vi "Dashboard Main for German stuff.vi"() -> ()   [LabVIEW 2013]
uses:
  <vilib>/Rock Robotics/WPI/DriverStation/WPI_DriverStationAllianceInfo.ctl
  <vilib>/Rock Robotics/WPI/Dashboard/WPI_DashboardLogging Global.vi
  <vilib>/Rock Robotics/WPI/Camera/WPI_CameraImageSize.ctl
  <vilib>/Rock Robotics/WPI/Camera/WPI_CameraSettings Read MJPG.ctl
panel:
  in  "Sudden Sound":bool
  in  "Oh Nein":bool
  out "Left Speed":dbl
  out "Right Speed":dbl
  in  "Precious":bool
  in  "Pokemon":bool
  in  "Yoda":bool
  in  "Alarm":bool
  in  "Scotty":bool
  in  "Hal":bool
  in  "Game over":bool
  in  "Gandalf":bool
  out "Teleop Time":dbl(slide) scale=0.0..150.0
  out "Right Power":dbl(slide) scale=-1.0..1.0
  out "Left Power":dbl(slide) scale=-1.0..1.0
  out "Shooter":u16(ring)
  out "Loader":u16(ring)
  out "Picture Information":u16(ring)
  in  "Camera view range":dbl=33.5 format="%#_13g"
  in  "Alliance 2":T1
  in  "Hot Side":dbl
  in  "Shooting Position Options":T2={TRUE, TRUE, TRUE, TRUE, TRUE, TRUE, TRUE, TRUE, TRUE, TRUE}
  out "Time Remaining":dbl(slide) scale=0.0..150.0
  in  "stop":bool
  out "Camera IP":string
  in  "DB Camera Config":bool
  out "Image Message":string="Timeout in Camera Communications"
  in  "Rec Mode":enum32{"Stop", "Record", "Playback"}(radio)
  out "Secondary Driver Camera":T3(plugin-control)
  out "Primary Driver Camera":T3(plugin-control)
  # "TeleOperated"
  # "Primary Driver Side"
  # "Secondary Driver Side"
  # "Autonomous"
  # "Checklist\n\n1: Is the robot plugged in?\n2: Is the robot turned on?\n3: Are the balls in the correct position?\n4: Set up Autonomous (shooting position options)"
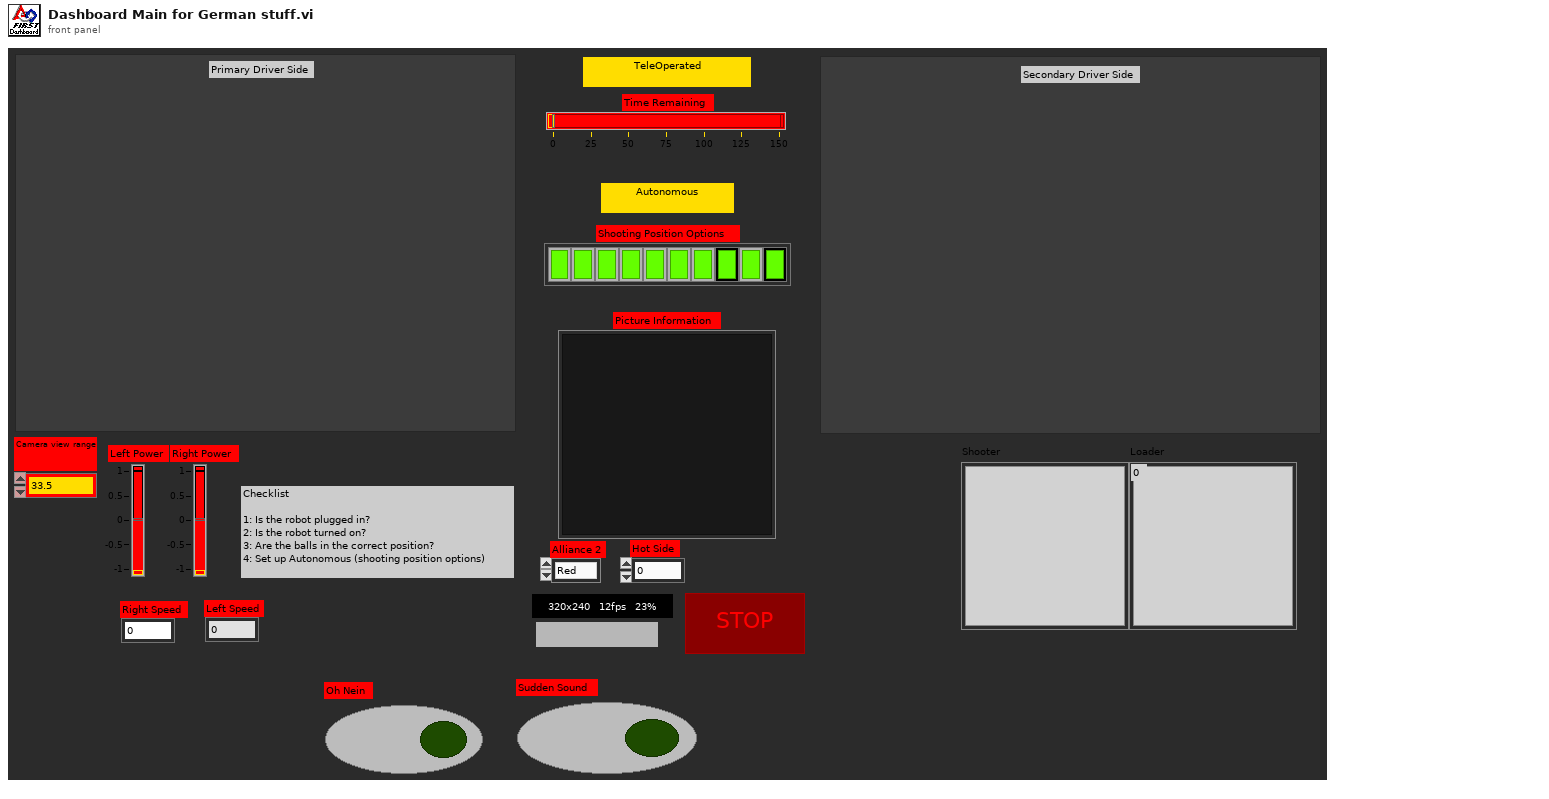
[diagram p1: front panel]
types:
  T1 = typedef "WPI_DriverStationAllianceInfo.ctl" = enum16{"Red", "Blue", "Invalid"}
  T2 = cluster{bool, bool, bool, bool, bool, bool, bool, bool, bool, bool}
  T3 = typedef "IMAQ Image.ctl" = refnum<image>
  T4 = cluster{"Left Power":dbl, "Right Power":dbl, "Shooter State":enum16{"Nothing", "Cocked", "Fire", "Load"}, "Loader State":enum16{"Loader Up", "Loader Down", "Ball In Possesion"}, "Auto Time":dbl, "Tele Time":dbl, "Driver":dbl, "Not Allowed":bool, "Right Speed":dbl, "Left Speed":dbl}
  T5 = enum16{"Loader Up", "Loader Down", "Ball In Possesion"}
  T6 = cluster{"Digital Inputs":bool[], "Digital Outputs":bool[]}
  T7 = cluster{"Competition mode":bool, "Robot Link":bool, "Autonomous":bool, "Enabled":bool, "E-Stop":bool, "Simulated":bool, "TestMode":bool, "Docked Window":bool}
  T8 = typedef "WPI_CameraSettings Read MJPG.ctl" = cluster{"fps":i32, "compression":i32, "Image Size":T9}
  T9 = typedef "WPI_CameraImageSize.ctl" = enum16{"640x480", "320x240", "160x120"}
  T10 = cluster{"Hue":dbl, "Saturation":dbl, "Luminance":dbl, "Hue Margin":dbl}
  T11 = typedef "Image Type" = u32
  T12 = cluster{"Left":i32, "Top":i32, "Right":i32, "Bottom":i32}
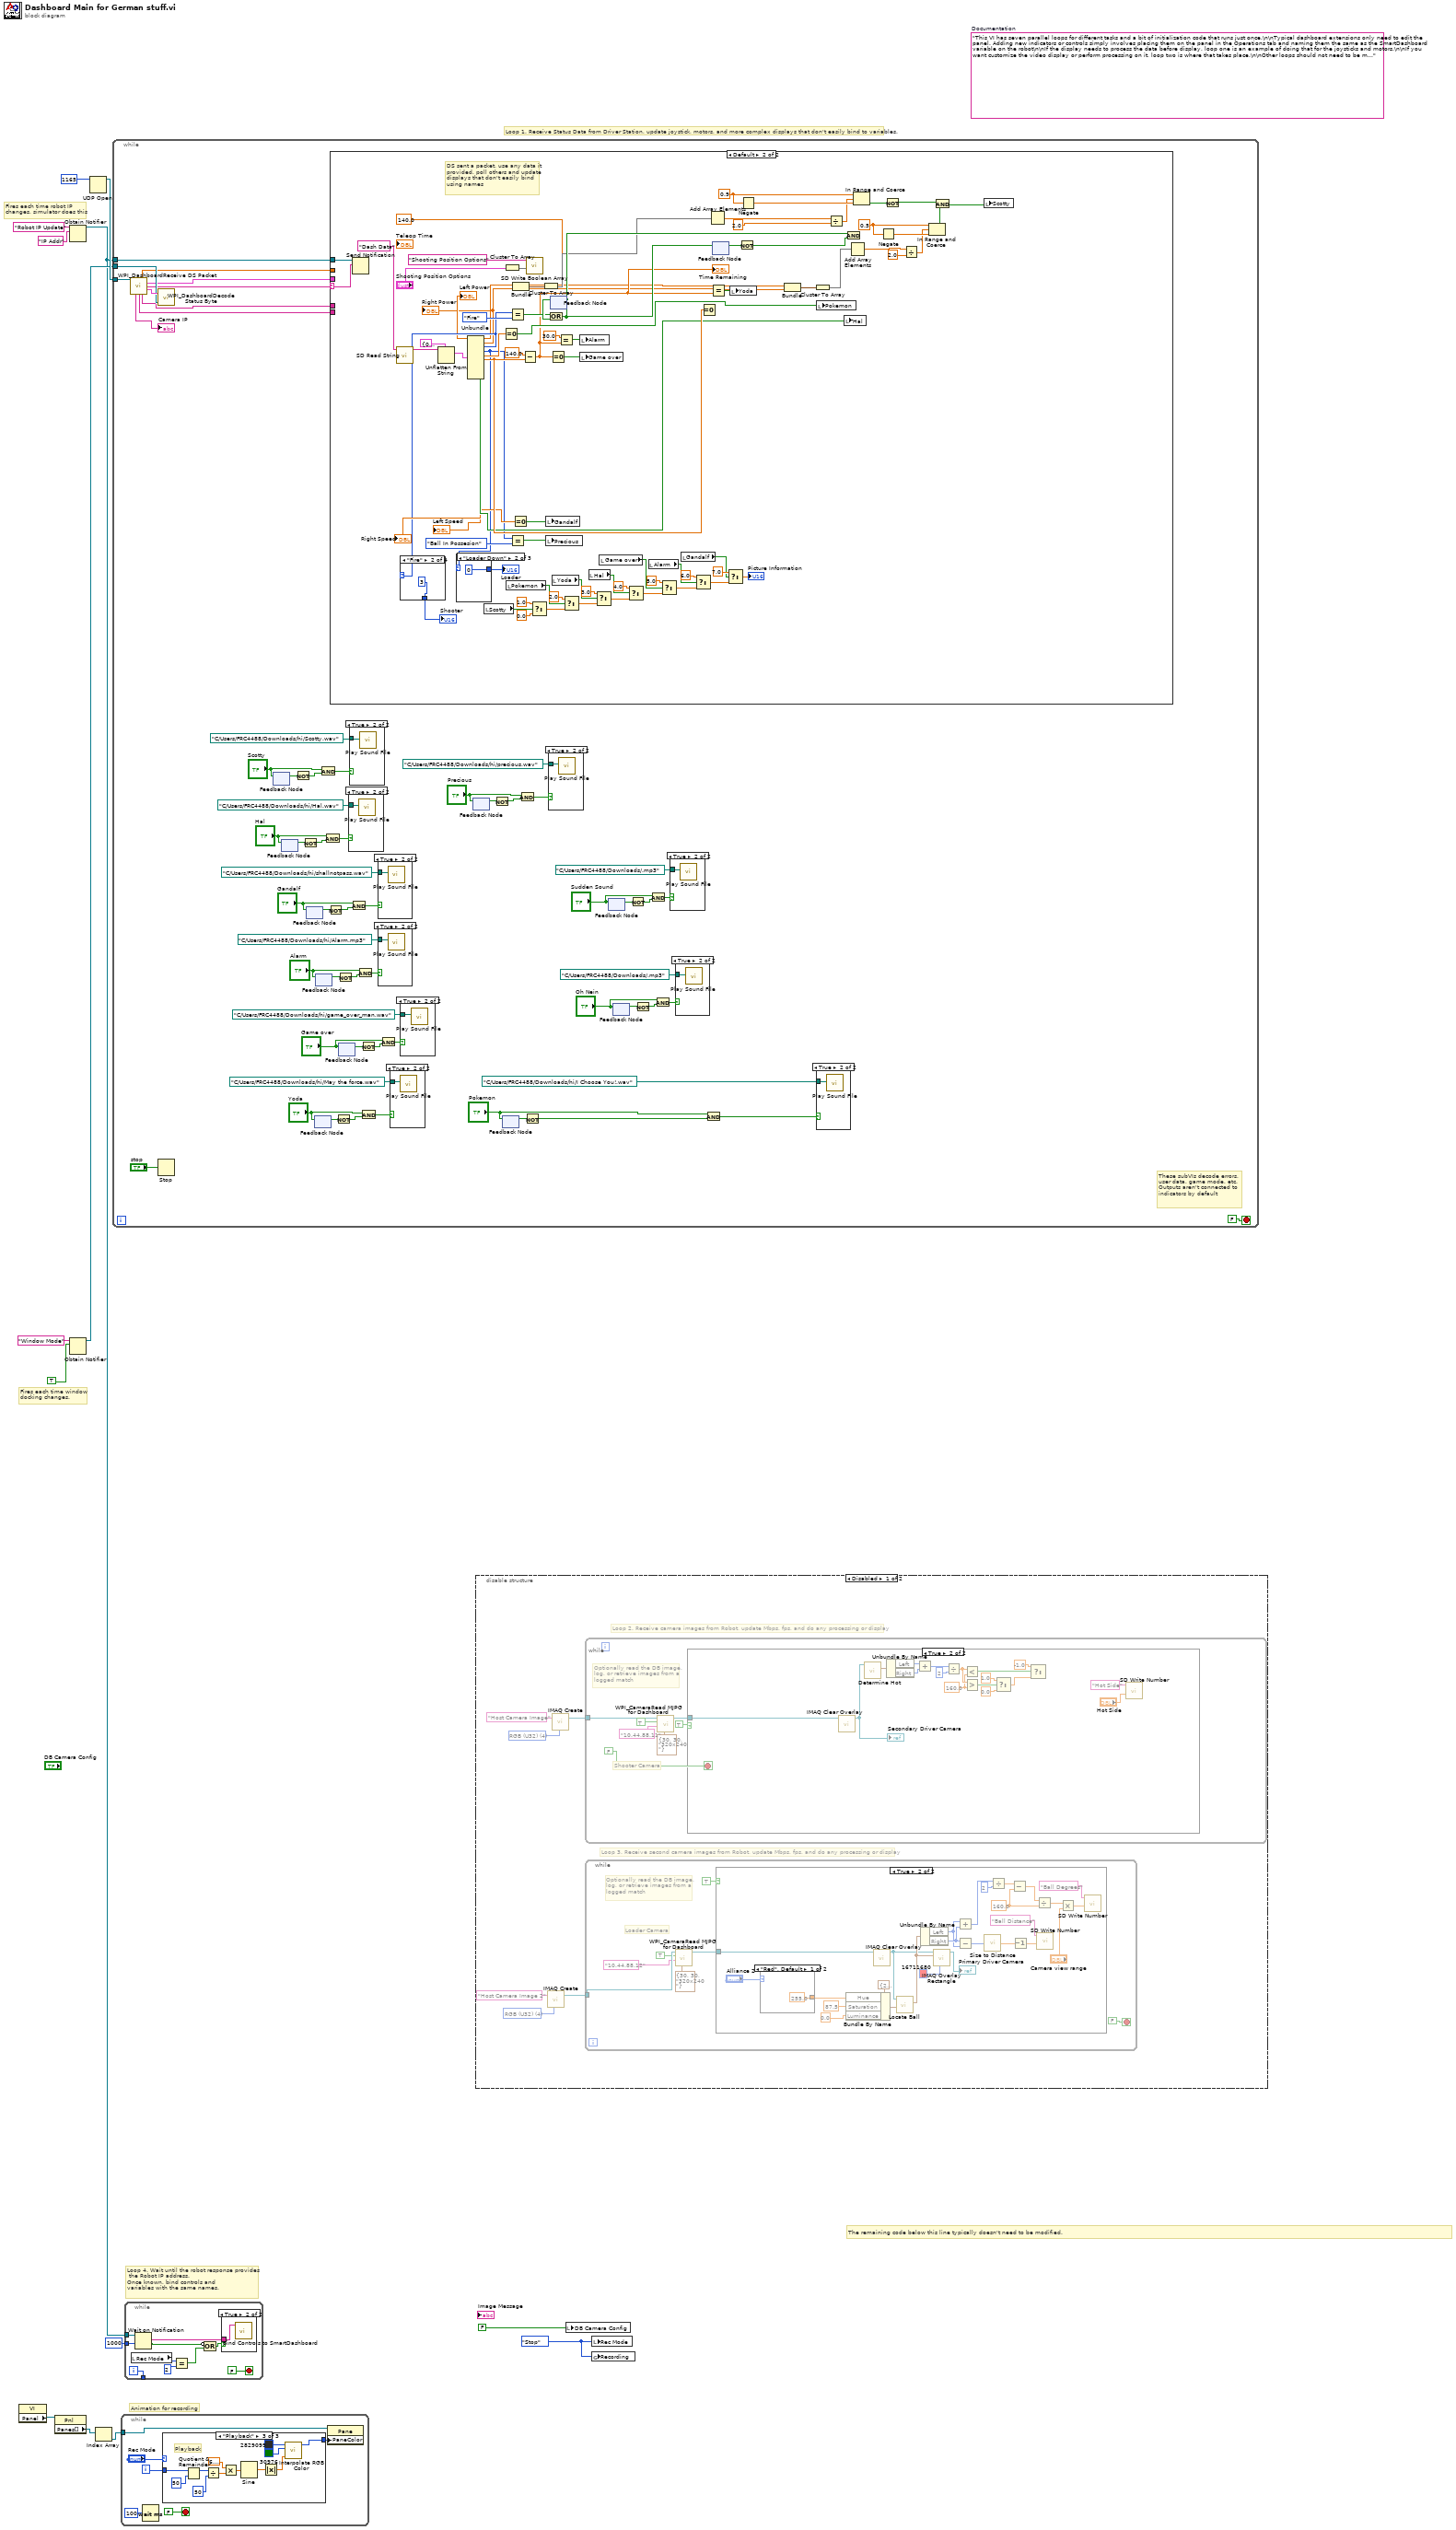
[diagram p0: block diagram]
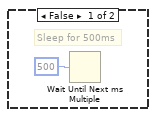
[diagram p2: hidden frame]
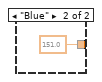
[diagram p3: hidden frame]
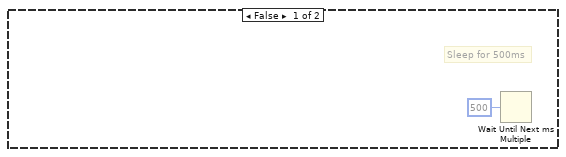
[diagram p4: hidden frame]
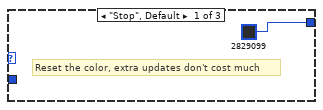
[diagram p6: hidden frame]
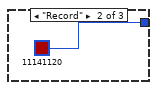
[diagram p7: hidden frame]
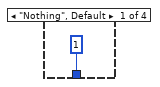
[diagram p20: hidden frame]
diagram:
  w2 = enum32{"Stop", "Record", "Playback"}."Stop" ("Rec Mode")
  (unwired) "This VI has seven parallel loops for different tasks and a bit of initialization code that runs just once.\n\nTypical dashboard extensions only need to edit the panel. Adding new indicators or controls simply involves placing them on the panel in the Operations tab and naming them the same as the SmartDashboard variable on the robot\n\nIf the display needs to process the data before display, loop one is an example of doing that for the joysticks and motors.\n\nIf you want customize the video display or perform processing on it, loop two is where that takes place.\n\nOther loops should not need to be modified. They are pretty standard, and document the task they perform."  # Documentation
  # "Animation for recording"
  # "Fires each time robot IP\nchanges, simulator does this"
  # "Fires each time window\ndocking changes."
  # "The remaining code below this line typically doesn't need to be modified."
  # "Loop 4. Wait until the robot response provides\n the Robot IP address.\nOnce known, bind controls and\nvariables with the same names."
  # "Loop 1. Receive Status Data from Driver Station, update joystick, motors, and more complex displays that don't easily bind to variables."
  n1 = property class="VI"() -> ("Panel"=w6:refnum<vi>)  [unwired: 2 in, 2 out]
  n2 = property class="Pnl"(reference=w6) -> ("Panes[]"=w7:refnum<vi>[])  [unwired: 1 in, 2 out]
  n3 = Obtain Notifier(name (unnamed)="Robot IP Update", notification data type="IP Addr" ("name (unnamed)")) -> (notifier out=w1:refnum<notifier>)  [unwired: 2 in, 2 out]
  n4 = Obtain Notifier(name (unnamed)="Window Mode", notification data type=TRUE) -> (notifier out=w3:refnum<notifier>)  [unwired: 2 in, 2 out]
  n5 = UDP Open(11:u16 1165 ("port")) -> (port=w13:refnum<k16>)  [unwired: 2 in, 4 out]
  n6 = Index Array(array=w7) -> (element=w5:refnum<vi>)  [unwired: 1 in]
  n7 = while {
    tunnel: w13 -> [w74]
    tunnel: w1 -> [w72]
    tunnel: w3 -> [w73]
    stop <- FALSE stop-if-true
    # "These subVIs decode errors, user data, game mode, etc.\nOutputs aren't connected to indicators by default"
    n8 = call <vilib>:"WPI_DashboardReceive DS Packet.vi"("Recv Socket"=w74) -> ("Battery"=w67:sgl, "Driver Station"=w68:T6, "Robot IP Address"=w71:string, "Status"=w75:T7, "Camera IP Address"=→"Camera IP":string, "Low Priority User Data"=w70:string, "High Priority User Data"=w69:string)  [unwired: 1 in, 7 out]
    n9 = call <vilib>:"WPI_DashboardDecode Status Byte.vi"("Window Mode Notifier"=w73, "Status"=w75) -> ()  [unwired: 2 out]
    n10 = Stop(stop? (T)="stop") -> ()
    n11 = feedback #1() -> (w52:bool)  [unwired: 1 in]
    n12 = feedback-in #1("Scotty") -> ()
    n13 = feedback #2() -> (w57:bool)  [unwired: 1 in]
    n14 = feedback-in #2("Hal") -> ()
    n15 = Not(x=w52) -> (.not. x?=w53:bool)
    n16 = Not(x=w57) -> (.not. x?=w56:bool)
    n17 = feedback #3() -> (w42:bool)  [unwired: 1 in]
    n18 = feedback-in #3("Gandalf") -> ()
    n19 = feedback #4() -> (w37:bool)  [unwired: 1 in]
    n20 = feedback-in #4("Yoda") -> ()
    n21 = feedback #5() -> (w47:bool)  [unwired: 1 in]
    n22 = feedback-in #5("Alarm") -> ()
    n23 = And(x="Scotty", y=w53) -> (x .and. y?=w50:bool)
    n24 = And(x="Hal", y=w56) -> (x .and. y?=w59:bool)
    n25 = Not(x=w42) -> (.not. x?=w41:bool)
    n26 = case shown="Default" w71 {
      selector: w71 -> [_ w163]
      tunnel: w72 -> [_ w164]
      tunnel: w70 -> [_ _]
      tunnel: w69 -> [_ _]
      tunnel: w68 -> [_ _]
      tunnel: w67 -> [_ _]
      frame "0.0.0.0" {
        # "DS not sending packets, or no robot exists yet.\nDon't poll the variables"
      }
      frame Default {
        w95 = 0.5 ("upper limit")
        w153 = 0.9 ("upper limit")
        # "DS sent a packet. use any data it\nprovided, poll others and update\ndisplays that don't easily bind\nusing names"
        n27 = Send Notification(notification=w163, notifier=w164) -> ()  [unwired: 1 in, 2 out]
        n28 = call <vilib>:"SD Read String.vi"("Name"="Dash Data") -> ("String"=w157:string)  [unwired: 8 in, 2 out]
        n29 = Unflatten From String(type=T4 {"Left Power"=0.0, "Right Power"=0.0, "Shooter State"=enum."Nothing", "Loader State"=enum."Loader Up", "Auto Time"=0.0, "Tele Time"=0.0, "Driver"=0.0, "Not Allowed"=FALSE, "Right Speed"=0.0, "Left Speed"=0.0} ("To Dashboard"), binary string=w157) -> (value=w145:T4)  [unwired: 3 in, 2 out]
        n30 = Unbundle(w145) -> ("Left Power"=w88:dbl, "Right Power"=w87:dbl, "Shooter State"=w100:enum16{"Nothing", "Cocked", "Fire", "Load"}, "Loader State"=w102:T5, "Auto Time"=w143:dbl, "Tele Time"=w144:dbl, "Driver"=w135:dbl, "Not Allowed"=w137:bool, "Right Speed"=→"Right Speed":dbl, "Left Speed"=→"Left Speed":dbl)
        "Left Power" <- w88
        "Right Power" <- w87
        n31 = case shown="\"Fire\"" w100 {
          tunnel: [1 3 2 0] -> w99
          frame "Nothing", Default {
          }
          frame "Fire" {
          }
          frame "Load" {
          }
          frame "Cocked" {
          }
        }
        "Shooter" <- w99
        n32 = case shown="\"Loader Down\"" w102 {
          tunnel: [1 0 2] -> w101
          frame "Loader Up", Default {
          }
          frame "Loader Down" {
          }
          frame "Ball In Possesion" {
          }
        }
        "Loader" <- w101
        n33 = local read "Scotty"() -> (w107:bool)
        n34 = Equal To 0?(x=w143) -> (x = 0?=w138:bool)
        n35 = Cluster To Array(cluster="Shooting Position Options") -> (array=w159:bool[])
        n36 = local read "Pokemon"() -> (w120:bool)
        n37 = Equal?(x=w100, y=enum16{"Nothing", "Fire", "Load"}."Fire") -> (x = y?=w141:bool)
        n38 = Equal?(x=w102, y=T5."Ball In Possesion" ("Loader State")) -> (x = y?=w129:bool)
        n39 = Equal To 0?(x=w135) -> (x = 0?=w136:bool)
        n40 = Bundle("Left Power"=w88, "Right Power"=w87) -> (w140:cluster{"Left Power":dbl, "Right Power":dbl})  [unwired: 1 in]
        n41 = Subtract(x=140.0, y=w144) -> (x-y=w133:dbl)
        "Time Remaining" <- w133
        n42 = call <vilib>:"SD Write Boolean Array.vi"("Boolean Array"=w159, "Name"="Shooting Position Options") -> ()  [unwired: 8 in, 2 out]
        n43 = Select(t=1.0, s=w107, f=0.0) -> (s? t:f=w111:dbl)
        n44 = Cluster To Array(cluster=w140) -> (array=w139:dbl[])
        n45 = local write "Gandalf"(w136) -> ()
        n46 = local write "Precious"(w129) -> ()
        n47 = Equal To 0?(x=w133) -> (x = 0?=w134:bool)
        n48 = feedback #6() -> (w149:bool)  [unwired: 1 in]
        n49 = Or(x=w141, y=w149) -> (x .or. y?=w148:bool)
        n50 = feedback-in #6(w148) -> ()
        n51 = local read "Yoda"() -> (w106:bool)
        n52 = Equal?(x=30.0, y=w133) -> (x = y?=w131:bool)
        n53 = Select(t=2.0, s=w120, f=w111) -> (s? t:f=w123:dbl)
        n54 = local write "Alarm"(w131) -> ()
        n55 = local write "Game over"(w134) -> ()
        n56 = local read "Hal"() -> (w119:bool)
        n57 = Select(t=3.0, s=w106, f=w123) -> (s? t:f=w124:dbl)
        n58 = local read "Game over"() -> (w118:bool)
        n59 = Select(t=4.0, s=w119, f=w124) -> (s? t:f=w125:dbl)
        n60 = local read "Alarm"() -> (w122:bool)
        n61 = Select(t=5.0, s=w118, f=w125) -> (s? t:f=w126:dbl)
        n62 = local read "Gandalf"() -> (w108:bool)
        n63 = Select(t=6.0, s=w122, f=w126) -> (s? t:f=w121:dbl)
        n64 = Equal To 0?(x=w144) -> ()  [unwired: 1 out]
        n65 = Add Array Elements(numeric array=w139) -> (sum=w156:dbl)
        n66 = Equal?(x=140.0, y=w133) -> (x = y?=w130:bool)
        n67 = feedback-in #7(w148) -> ()
        n68 = feedback #7() -> (w147:bool)  [unwired: 1 in]
        n69 = Select(t=7.0, s=w108, f=w121) -> (s? t:f=→"Picture Information":dbl)
        n70 = local write "Yoda"(w130) -> ()
        n71 = Not(x=w147) -> (.not. x?=w146:bool)
        n72 = Negate(x=w153) -> (-x=w154:dbl)
        n73 = Bundle("Left Power"=w88, "Right Power"=w87) -> (w92:cluster{"Left Power":dbl, "Right Power":dbl})  [unwired: 1 in]
        n74 = Cluster To Array(cluster=w92) -> (array=w91:dbl[])
        n75 = local write "Pokemon"(w138) -> ()
        n76 = Divide(x=w156, y=2.0) -> (x/y=w152:dbl)
        n77 = local write "Hal"(w137) -> ()
        n78 = And(x=w148, y=w146) -> ()  [unwired: 1 out]
        n79 = Add Array Elements(numeric array=w91) -> (sum=w90:dbl)
        n80 = In Range and Coerce(upper limit=w153, x=w152, lower limit=w154) -> (In Range?=w151:bool)  [unwired: 1 out]
        n81 = Negate(x=w95) -> (-x=w96:dbl)
        n82 = Not(x=w151) -> (.not. x?=w98:bool)
        n83 = Divide(x=w90, y=2.0) -> (x/y=w94:dbl)
        n84 = In Range and Coerce(upper limit=w95, x=w94, lower limit=w96) -> (In Range?=w89:bool)  [unwired: 1 out]
        n85 = And(x=w98, y=w89) -> (x .and. y?=w97:bool)
        n86 = local write "Scotty"(w97) -> ()
      }
    }
    n87 = Not(x=w37) -> (.not. x?=w38:bool)
    n88 = Not(x=w47) -> (.not. x?=w48:bool)
    n89 = feedback #8() -> (w62:bool)  [unwired: 1 in]
    n90 = feedback-in #8("Game over") -> ()
    n91 = case shown="True" w59 {
      tunnel: path "C:/Users/FRC4488/Downloads/hi/Hal.wav" ("path") -> [_ w85]
      frame False {
      }
      frame True {
        n92 = call <vilib>:"Play Sound File.vi"("path"=w85) -> ()  [unwired: 9 in, 2 out]
      }
    }
    n93 = case shown="True" w50 {
      tunnel: path "C:/Users/FRC4488/Downloads/hi/Scotty.wav" ("path") -> [_ w84]
      frame False {
      }
      frame True {
        n94 = call <vilib>:"Play Sound File.vi"("path"=w84) -> ()  [unwired: 9 in, 2 out]
      }
    }
    n95 = And(x="Gandalf", y=w41) -> (x .and. y?=w44:bool)
    n96 = And(x="Alarm", y=w48) -> (x .and. y?=w45:bool)
    n97 = Not(x=w62) -> (.not. x?=w63:bool)
    n98 = And(x="Yoda", y=w38) -> (x .and. y?=w35:bool)
    n99 = case shown="True" w44 {
      tunnel: path "C:/Users/FRC4488/Downloads/hi/shallnotpass.wav" ("path") -> [_ w82]
      frame False {
      }
      frame True {
        n100 = call <vilib>:"Play Sound File.vi"("path"=w82) -> ()  [unwired: 9 in, 2 out]
      }
    }
    n101 = case shown="True" w45 {
      tunnel: path "C:/Users/FRC4488/Downloads/hi/Alarm.mp3" ("path") -> [_ w83]
      frame False {
      }
      frame True {
        n102 = call <vilib>:"Play Sound File.vi"("path"=w83) -> ()  [unwired: 9 in, 2 out]
      }
    }
    n103 = And(x="Game over", y=w63) -> (x .and. y?=w60:bool)
    n104 = case shown="True" w35 {
      tunnel: path "C:/Users/FRC4488/Downloads/hi/May the force.wav" ("path") -> [_ w81]
      frame False {
      }
      frame True {
        n105 = call <vilib>:"Play Sound File.vi"("path"=w81) -> ()  [unwired: 9 in, 2 out]
      }
    }
    n106 = case shown="True" w60 {
      tunnel: path "C:/Users/FRC4488/Downloads/hi/game_over_man.wav" ("path") -> [_ w86]
      frame False {
      }
      frame True {
        n107 = call <vilib>:"Play Sound File.vi"("path"=w86) -> ()  [unwired: 9 in, 2 out]
      }
    }
    n108 = feedback #9() -> (w27:bool)  [unwired: 1 in]
    n109 = feedback-in #9("Precious") -> ()
    n110 = Not(x=w27) -> (.not. x?=w28:bool)
    n111 = feedback #10() -> (w31:bool)  [unwired: 1 in]
    n112 = feedback-in #10("Pokemon") -> ()
    n113 = And(x="Precious", y=w28) -> (x .and. y?=w25:bool)
    n114 = Not(x=w31) -> (.not. x?=w32:bool)
    n115 = case shown="True" w25 {
      tunnel: path "C:/Users/FRC4488/Downloads/hi/precious.wav" ("path") -> [_ w79]
      frame False {
      }
      frame True {
        n116 = call <vilib>:"Play Sound File.vi"("path"=w79) -> ()  [unwired: 9 in, 2 out]
      }
    }
    n117 = feedback #11() -> (w17:bool)  [unwired: 1 in]
    n118 = feedback-in #11("Sudden Sound") -> ()
    n119 = feedback #12() -> (w22:bool)  [unwired: 1 in]
    n120 = feedback-in #12("Oh Nein") -> ()
    n121 = Not(x=w17) -> (.not. x?=w18:bool)
    n122 = Not(x=w22) -> (.not. x?=w21:bool)
    n123 = And(x="Sudden Sound", y=w18) -> (x .and. y?=w15:bool)
    n124 = And(x="Oh Nein", y=w21) -> (x .and. y?=w24:bool)
    n125 = case shown="True" w15 {
      tunnel: path "C:/Users/FRC4488/Downloads/.mp3" ("path") -> [_ w77]
      frame False {
      }
      frame True {
        n126 = call <vilib>:"Play Sound File.vi"("path"=w77) -> ()  [unwired: 9 in, 2 out]
      }
    }
    n127 = case shown="True" w24 {
      tunnel: path "C:/Users/FRC4488/Downloads/.mp3" ("path") -> [_ w78]
      frame False {
      }
      frame True {
        n128 = call <vilib>:"Play Sound File.vi"("path"=w78) -> ()  [unwired: 9 in, 2 out]
      }
    }
    n129 = And(x="Pokemon", y=w32) -> (x .and. y?=w34:bool)
    n130 = case shown="True" w34 {
      tunnel: path "C:/Users/FRC4488/Downloads/hi/I Choose You!.wav" ("path") -> [_ w80]
      frame False {
      }
      frame True {
        n131 = call <vilib>:"Play Sound File.vi"("path"=w80) -> ()  [unwired: 9 in, 2 out]
      }
    }
  }
  n132 = while {
    tunnel: w5 -> [w173]
    i -> [w176]
    stop <- FALSE stop-if-true
    n133 = Wait (ms)(milliseconds to wait=u32 100) -> ()  [unwired: 1 out]
    n134 = case shown="\"Playback\"" "Rec Mode" {
      tunnel: w176 -> [_ _ w191]
      tunnel: [u32 2829099 ("Base Color") u32 11141120 ("Target Color") w180] -> w172
      frame "Stop", Default {
        # "Reset the color, extra updates don't cost much"
      }
      frame "Record" {
      }
      frame "Playback" {
        # "Playback"
        n135 = Quotient & Remainder(x=w191, y=u32 50 ("milliseconds to wait")) -> (x-y*floor(x/y)=w187:u32)  [unwired: 1 out]
        n136 = Divide(x=w187, y=u32 50 ("milliseconds to wait")) -> (x/y=w184:dbl)
        n137 = Multiply(x=6.283185307179586, y=w184) -> (x*y=w189:dbl)
        n138 = Sine(x=w189) -> (sin(x)=w188:dbl)
        n139 = Absolute Value(x=w188) -> (abs(x)=w181:dbl)
        n140 = call "Interpolate RGB Color.vi"("Proportion"=w181, "Target Color"=u32 30976, "Base Color"=u32 2829099) -> ("Result Color"=w180:u32)  [unwired: 8 in]
      }
    }
    n141 = property class="Pane"(reference=w173, "PaneColor"=w172) -> ()  [unwired: 1 in, 2 out]
  }
  n142 = while {
    tunnel: w1 -> [w200]
    tunnel: [w198] -> _
    tunnel: u32 1000 ("milliseconds to wait") -> [w197]
    i -> [w198]
    stop <- FALSE stop-if-true
    n143 = local read "Rec Mode"() -> (w193:enum32{"Stop", "Record", "Playback"})
    n144 = Wait on Notification(notifier=w200, timeout in ms (-1)=w197) -> (notification=w199:string, timed out?=w195:bool)  [unwired: 2 in, 2 out]
    n145 = Equal?(x=w193, y=u16 2 ("Rec Mode")) -> (x = y?=w194:bool)
    n146 = Compound Arithmetic op=OR(invert w195, w194) -> (w196:bool)
    n147 = case shown="True" w196 {
      tunnel: w199 -> [_ w202]
      frame False {
      }
      frame True {
        n148 = call <vilib>:"Bind Controls to SmartDashboard.vi"("Server IP Address"=w202) -> ()  [unwired: 11 in]
      }
    }
  }
  n149 = disable-structure shown="Disabled" {
    frame Disabled {
      w203 = T11 4 items=["Grayscale (U8)", "Grayscale (I16)", "Grayscale (SGL)", "Complex (CSG)", "RGB (U32)", "HSL (U32)", "RGB (U64)"] ("Image Type")
      w208 = T11 4 items=["Grayscale (U8)", "Grayscale (I16)", "Grayscale (SGL)", "Complex (CSG)", "RGB (U32)", "HSL (U32)", "RGB (U64)"] ("Image Type")
      # "Loop 3. Receive second camera images from Robot, update Mbps, fps, and do any processing or display"
      # "Loop 2. Receive camera images from Robot, update Mbps, fps, and do any processing or display"
      n150 = call "IMAQ Create"("Image Name"="Host Camera Image 2", "Image Type"=w203) -> ("New Image"=w205:T3)  [unwired: 2 in, 2 out]
      n151 = call "IMAQ Create"("Image Name"="Host Camera Image", "Image Type"=w208) -> ("New Image"=w206:T3)  [unwired: 2 in, 2 out]
      n152 = while {
        tunnel: w205 -> [w214]
        stop <- FALSE stop-if-true
        # "Loader Camera"
        # "Optionally read the DB image,\nlog, or retrieve images from a\nlogged match"
        n153 = call <vilib>:"WPI_CameraRead MJPG for Dashboard.vi"("Camera Settings"=T8 {"fps"=30, "compression"=30, "Image Size"=enum."320x240"}, "Camera IP"="10.44.88.12", "Enable"=TRUE ("Enable 2"), "Refnum in"=w214) -> ("Refnum out"=w213:T3)  [unwired: 4 in, 3 out]
        n154 = case shown="True" TRUE ("Enable 2") {
          tunnel: w213 -> [_ w242]
          frame False {
            # "Sleep for 500ms"
            n155 = Wait Until Next ms Multiple(millisecond multiple=u32 500) -> ()  [unwired: 1 out]
          }
          frame True {
            w237 = 160.0 ("y")
            n156 = case shown="\"Red\", Default" "Alliance 2" {
              tunnel: [255.0 ("Hue") 151.0 ("Hue")] -> w223
              frame "Red", Default {
              }
              frame "Blue" {
              }
            }
            n157 = Bundle By Name(cluster=T10 {"Hue"=254.37461497254125, "Saturation"=85.0, "Luminance"=0.0, "Hue Margin"=40.0} ("Hue Selector"), "Hue"=w223, "Saturation"=87.5, "Luminance"=0.0) -> (w220:T10)
            n158 = call "IMAQ Clear Overlay"("Image"=w242) -> ("Image Out"=w225:T3)  [unwired: 2 in, 8 out]
            n159 = call "Locate Ball.vi"("New Image"=w225, "Hue Selector"=w220) -> ("Rectangle"=w231:T12)  [unwired: 7 in, 1 out]
            n160 = Unbundle By Name(w231) -> ("Left"=w233:i32, "Right"=w234:i32)
            n161 = call "IMAQ Overlay Rectangle"("Color"=u32 16711680, "Rectangle"=w231, "Image"=w225) -> ("Image Out"=→"Primary Driver Camera":T3)  [unwired: 7 in, 1 out]
            n162 = Add(x=w233, y=w234) -> (x+y=w241:i32)
            n163 = Subtract(x=w234, y=w233) -> (x-y=w228:i32)
            n164 = call "Size to Distance.vi"("Numeric"=w228) -> ("Numeric 2"=w227:dbl)
            n165 = Divide(x=w241, y=2) -> (x/y=w239:dbl)
            n166 = Subtract(x=w239, y=w237) -> (x-y=w238:dbl)
            n167 = Decrement(x=w227) -> (x-1=w226:dbl)
            n168 = Divide(x=w238, y=w237) -> (x/y=w236:dbl)
            n169 = call <vilib>:"SD Write Number.vi"("Numeric"=w226, "Name"="Ball Distance") -> ()  [unwired: 8 in, 2 out]
            n170 = Multiply(x=w236, y="Camera view range") -> (x*y=w229:dbl)
            n171 = call <vilib>:"SD Write Number.vi"("Numeric"=w229, "Name"="Ball Degrees") -> ()  [unwired: 8 in, 2 out]
          }
        }
      }
      n172 = while {
        tunnel: w206 -> [w250]
        stop <- FALSE stop-if-true
        # "Shooter Camera"
        # "Optionally read the DB image,\nlog, or retrieve images from a\nlogged match"
        n173 = call <vilib>:"WPI_CameraRead MJPG for Dashboard.vi"("Camera Settings"=T8 {"fps"=30, "compression"=30, "Image Size"=enum."320x240"}, "Camera IP"="10.44.88.11", "Enable"=TRUE ("Enable 2"), "Refnum in"=w250) -> ("Refnum out"=w249:T3)  [unwired: 4 in, 3 out]
        n174 = case shown="True" TRUE ("Enable 2") {
          tunnel: w249 -> [_ w269]
          frame False {
            # "Sleep for 500ms"
            n175 = Wait Until Next ms Multiple(millisecond multiple=u32 500) -> ()  [unwired: 1 out]
          }
          frame True {
            w258 = 160.0 ("y")
            n176 = call "IMAQ Clear Overlay"("Image"=w269) -> ("Image Out"=w253:T3)  [unwired: 2 in, 8 out]
            "Secondary Driver Camera" <- w253
            n177 = call "Determine Hot.vi"("New Image"=w253) -> ("Rectangle"=w268:T12)  [unwired: 8 in, 1 out]
            n178 = Unbundle By Name(w268) -> ("Left"=w265:i32, "Right"=w264:i32)
            n179 = Add(x=w265, y=w264) -> (x+y=w262:i32)
            n180 = Divide(x=w262, y=2) -> (x/y=w259:dbl)
            n181 = Less?(x=w259, y=w258) -> (x < y?=w261:bool)
            n182 = Greater?(x=w259, y=w258) -> (0:w257:bool)
            n183 = Select(t=1.0, s=w257, f=0.0) -> (s? t:f=w255:dbl)
            n184 = Select(t=-1.0, s=w261, f=w255) -> ()  [unwired: 1 out]
            n185 = call <vilib>:"SD Write Number.vi"("Numeric"="Hot Side", "Name"="Hot Side") -> ()  [unwired: 8 in, 2 out]
          }
        }
      }
    }
    frame Enabled {
    }
  }
  n186 = local write "DB Camera Config"(FALSE ("Visible")) -> ()
  n187 = local write "Rec Mode"(w2) -> ()
  n188 = global write "WPI_DashboardLogging Global.vi" "Recording"(w2) -> ()
